vi "Convert Position Units to Device Units.vi"(9 "Microstep Size (0)":dbl, 10 "Units (0: microsteps)":u16(ring) items=["microsteps", "microns", "millimeters", "inches", "degrees"], 11 "Position (0)":dbl) -> (1 "Device Position (64-bit)":i64, 2 "Device Position (String)":string, 3 "Device Position (32-bit)":i32)   [LabVIEW 2020, in "Zaber A Series.lvlib"]
doc: "Helper to convert standard units of measure to device-specific position units.\n\nSelect a unit and enter a Position quantity, which can be an absolute position or a relative position, and select a unit to convert from. \n\nIf you select a unit other than microsteps, you must also provide the Microstep Size conversion factor from microsteps to micrometers (for linear devices) or degrees (for rotary devices), which can be found in your device manual."
uses:
  Zaber A Series.lvlib
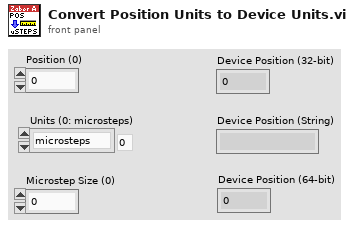
[diagram p1: front panel]
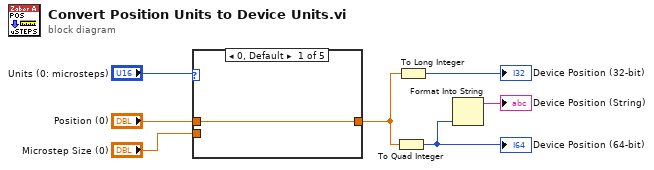
[diagram p0: block diagram]
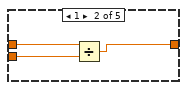
[diagram p2: hidden frame]
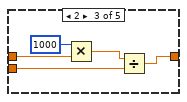
[diagram p3: hidden frame]
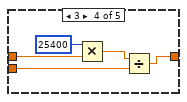
[diagram p4: hidden frame]
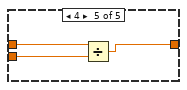
[diagram p5: hidden frame]
diagram:
  n1 = case shown="0, Default" "Units (0: microsteps)" {
    tunnel: "Position (0)" -> [w8 w11 w16 w19 w24]
    tunnel: "Microstep Size (0)" -> [_ w10 w13 w18 w23]
    tunnel: [w8 w9 w12 w17 w22] -> w3
    frame 0, Default {
    }
    frame 1 {
      n2 = Divide(x=w11, y=w10) -> (x/y=w9:dbl)
    }
    frame 2 {
      n3 = Multiply(x=1000, y=w16) -> (x*y=w14:dbl)
      n4 = Divide(x=w14, y=w13) -> (x/y=w12:dbl)
    }
    frame 3 {
      n5 = Multiply(x=25400, y=w19) -> (x*y=w20:dbl)
      n6 = Divide(x=w20, y=w18) -> (x/y=w17:dbl)
    }
    frame 4 {
      n7 = Divide(x=w24, y=w23) -> (x/y=w22:dbl)
    }
  }
  n8 = To Quad Integer(1:w3) -> (0:w2:i64)
  "Device Position (64-bit)" <- w2
  n9 = To Long Integer(number=w3) -> (32bit integer=→"Device Position (32-bit)":i32)
  n10 = Format Into String(w2) -> (resulting string=→"Device Position (String)":string)  [unwired: 3 in, 1 out]
